vi "Get Test Name.vi"(8 "error in (no error)":errorcluster, 11 "Assertion Result In":refnum<class "Assertion Result.lvclass">) -> (0 "error out":errorcluster, 2 "Message":string, 3 "Assertion Result Out":refnum<class "Assertion Result.lvclass">)   [LabVIEW 2020, in "Assertion Result.lvclass"]
uses:
  Assertion Result.lvclass
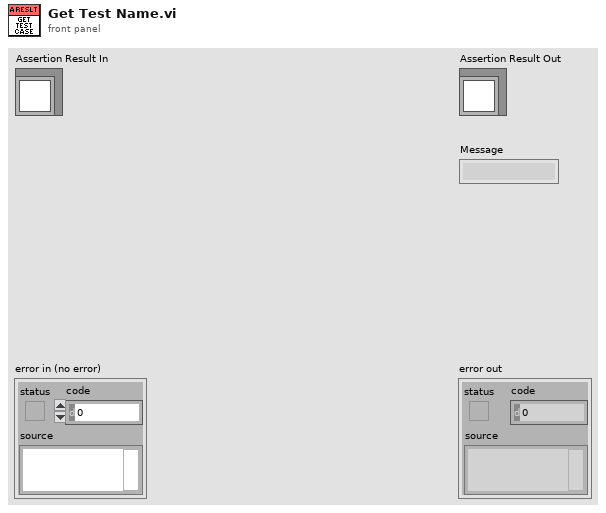
[diagram p1: front panel]
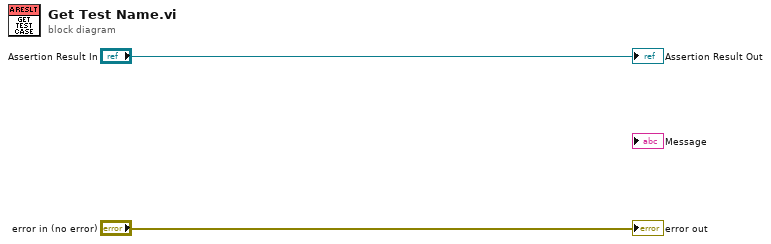
[diagram p0: block diagram]
diagram:
  "error out" <- "error in (no error)"
  "Assertion Result Out" <- "Assertion Result In"
